vi "test_section_daqmx_task.vi"(8 "error in":errorcluster, 9 "Test Section Physical Channels":T1={"Vapor Mass Flow Current"="cDAQ1Mod1/ai10", "Vapor Line Density Current"="cDAQ1Mod1/ai11", "Liquid Mass Flow Current"="cDAQ1Mod1/ai8", "Liquid Line Density Current"="cDAQ1Mod1/ai9", "Vapor Tank Pressure"="cDAQ1Mod1/ai3", "Liquid Tank Pressure"="cDAQ1Mod1/ai6", "Separator Pressure"="cDAQ1Mod1/ai2", "Liquid Inlet Pressure"="cDAQ1Mod1/ai4", "Dev Section Pressure"="cDAQ1Mod1/ai0", "Vapor Tank Temperature"="cDAQ1Mod1/ai1", "Vapor Inlet Temperature"="cDAQ1Mod6/ai2", "Liquid Tank Temperature"="cDAQ1Mod6/ai0", "Liquid Inlet Temperature"="cDAQ1Mod6/ai3", "Separator Temperature"="cDAQ1Mod6/ai4", "Lower Test Section Pressure"="cDAQ1Mod6/ai1", "Lower Test Section Temperature"="cDAQ1Mod1/ai5", "Top Heater Temperature"="cDAQ1Mod6/ai5", "Bottom Heater Temperature"="cDAQ1Mod6/ai6", "Pressure Drop"="cDAQ1Mod1/ai12", "Upper Test Section Temperature"="cDAQ1Mod1/ai12", "Upper Test Section Pressure"="cDAQ1Mod6/ai9", "Condenser Top Temperature"="cDAQ1Mod1/ai7", "Condenser Bottom Temperature"="cDAQ1Mod6/ai8", "Evaporator Top Temperature"="cDAQ1Mod6/ai10", "Evaporator Bottom Temperature"="cDAQ1Mod6/ai11", "Test Section Window 3-4 Pressure"="cDAQ1Mod6/ai12"}, 10 "sampling rate":dbl, 11 "number of samples":i32) -> (0 "error out":errorcluster, 3 "task out":refnum<k21>)   [LabVIEW 2015]
uses:
  <vilib>/DAQmx/create/channels.llb/DAQmx Create Channel (TEDS-AI-Current-Basic).vi
  <vilib>/DAQmx/create/channels.llb/DAQmx Create Channel (AI-Current-Basic).vi
  <vilib>/DAQmx/create/channels.llb/DAQmx Create Channel (AI-Voltage-Basic).vi
  <vilib>/DAQmx/create/channels.llb/DAQmx Create Channel (TEDS-AI-Voltage-Basic).vi
  <vilib>/DAQmx/create/channels.llb/DAQmx Create Channel (TEDS-AI-Temperature-Thermocouple).vi
  <vilib>/DAQmx/create/channels.llb/DAQmx Create Channel (AI-Temperature-Thermocouple).vi
  <resource>/objmgr/daqmx.rc
  <vilib>/DAQmx/configure/timing.llb/DAQmx Timing (Sample Clock).vi
  Input Channel Lists/test_section_physical_channels.ctl
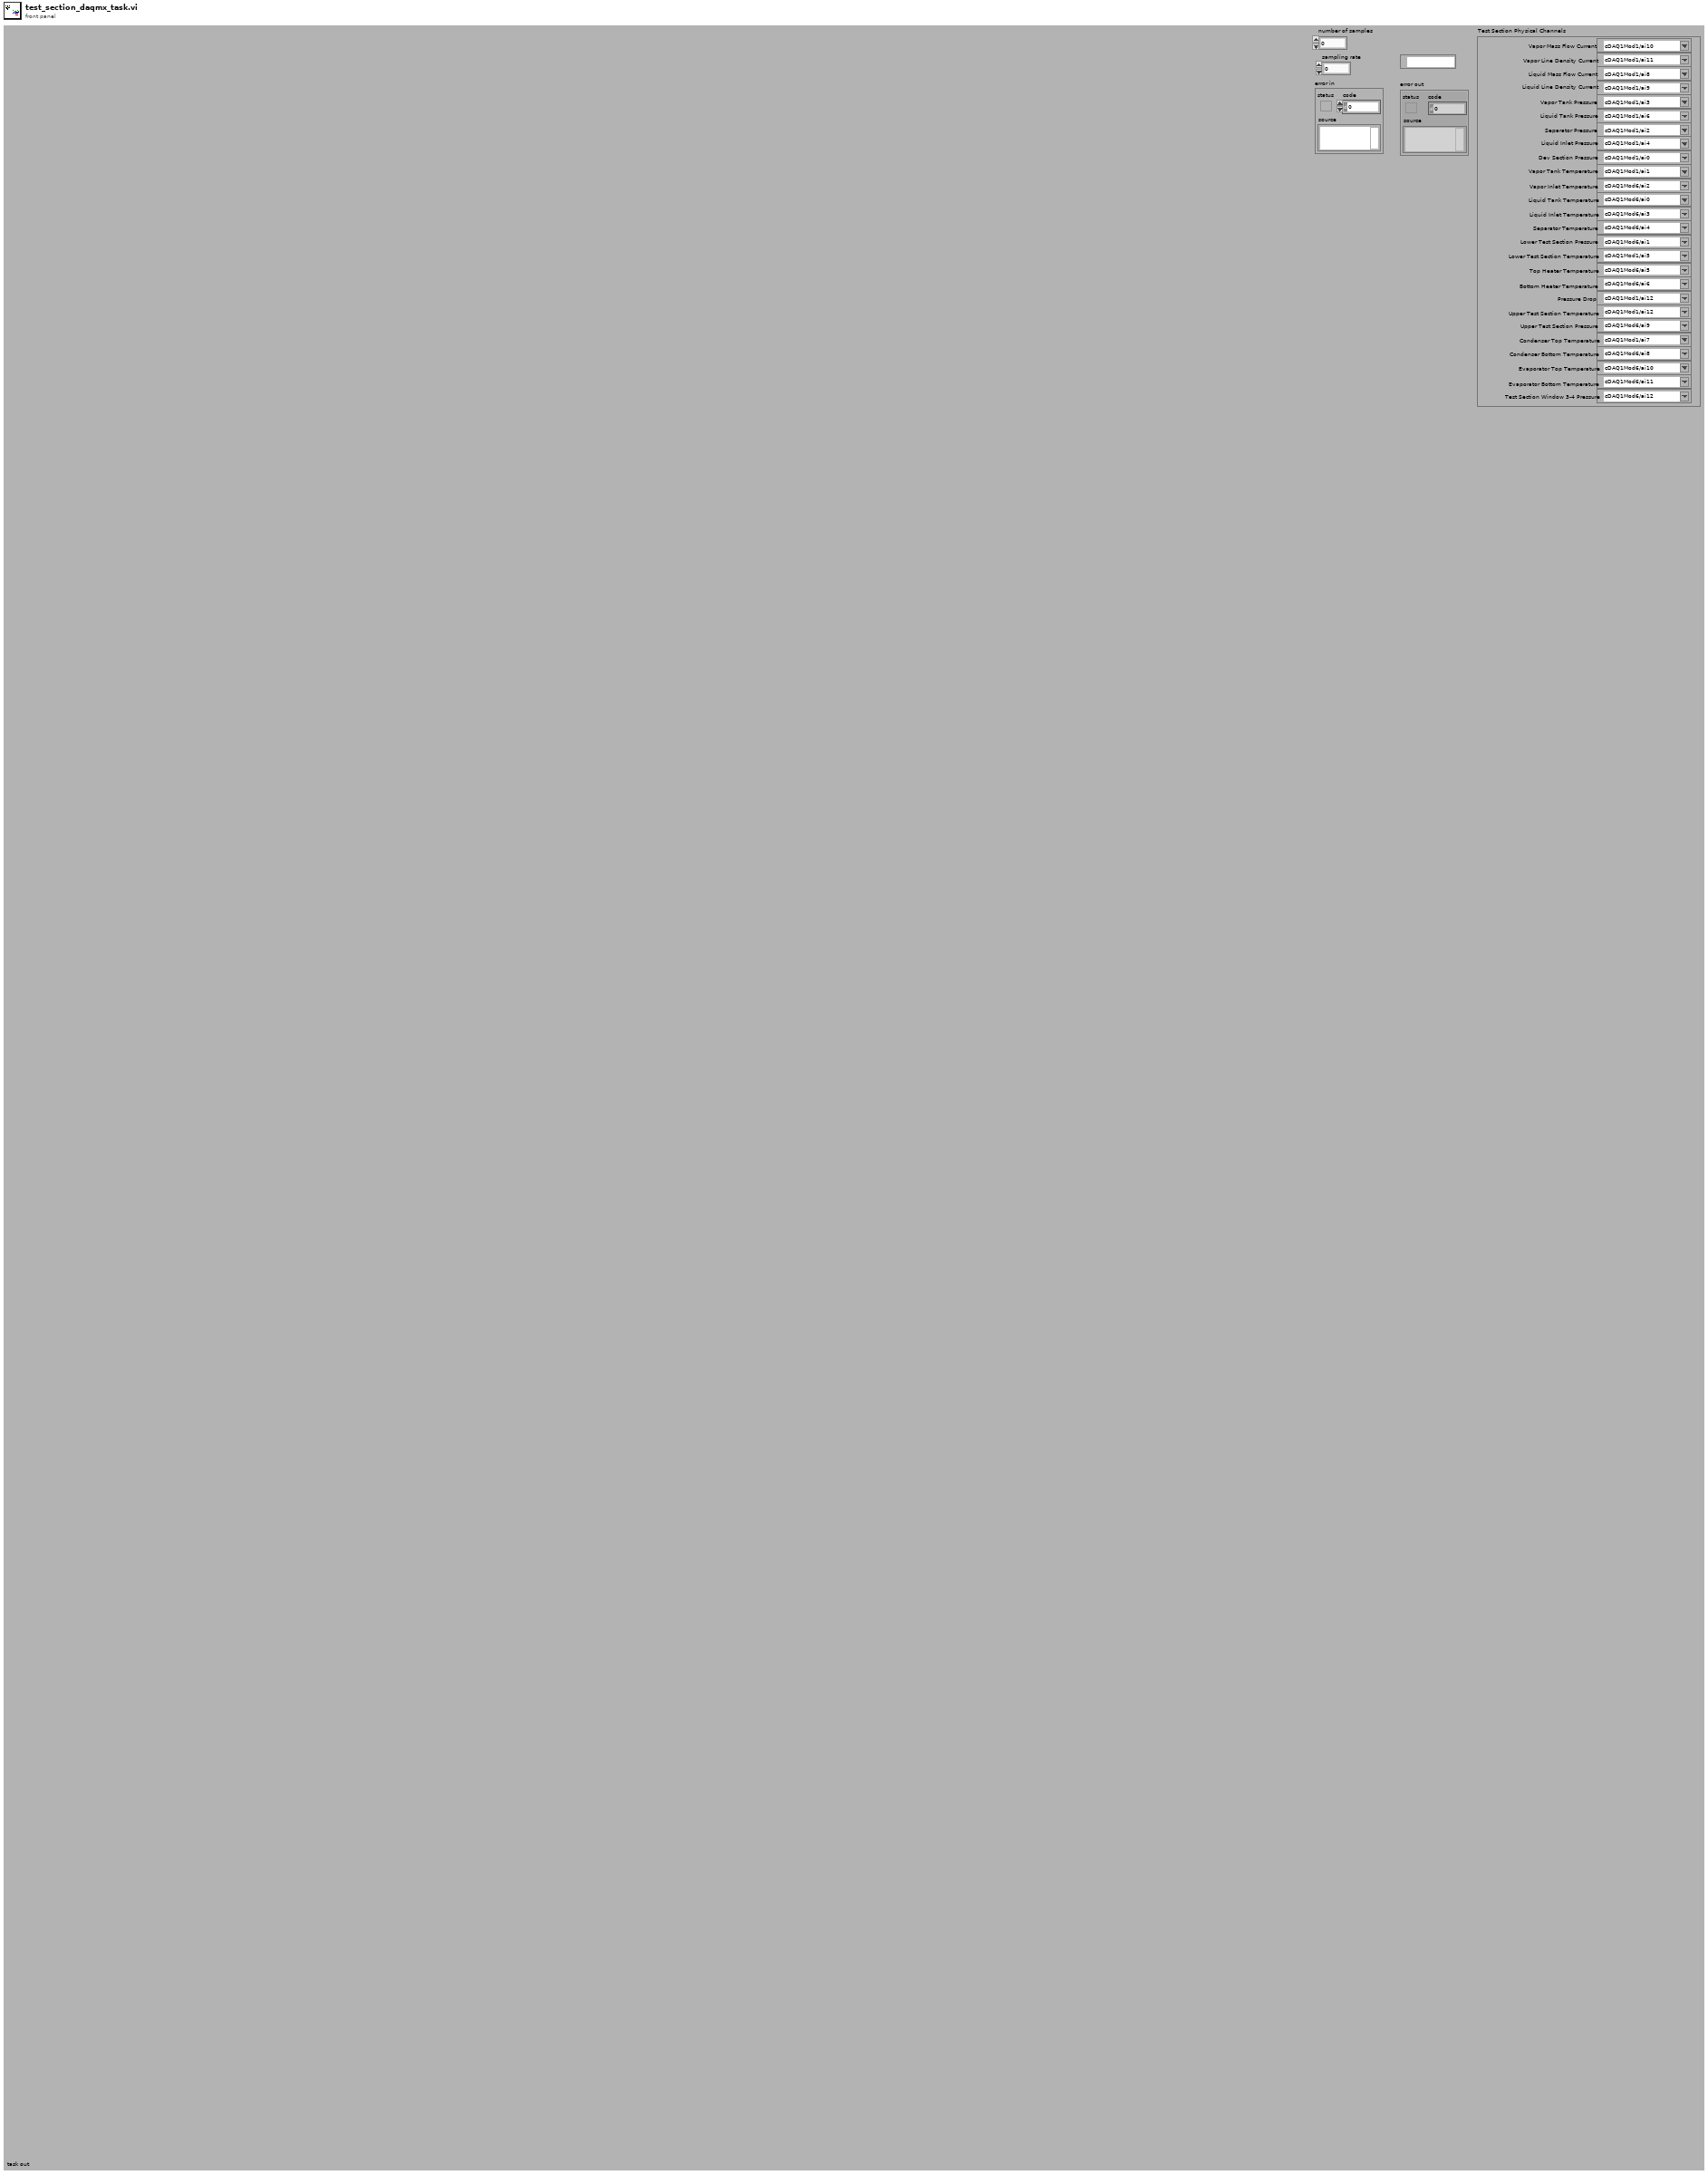
[diagram p1: front panel]
types:
  T1 = typedef "test_section_physical_channels.ctl" = cluster{"Vapor Mass Flow Current":tag, "Vapor Line Density Current":tag, "Liquid Mass Flow Current":tag, "Liquid Line Density Current":tag, "Vapor Tank Pressure":tag, "Liquid Tank Pressure":tag, "Separator Pressure":tag, "Liquid Inlet Pressure":tag, "Dev Section Pressure":tag, "Vapor Tank Temperature":tag, "Vapor Inlet Temperature":tag, "Liquid Tank Temperature":tag, "Liquid Inlet Temperature":tag, "Separator Temperature":tag, "Lower Test Section Pressure":tag, "Lower Test Section Temperature":tag, "Top Heater Temperature":tag, "Bottom Heater Temperature":tag, "Pressure Drop":tag, "Upper Test Section Temperature":tag, "Upper Test Section Pressure":tag, "Condenser Top Temperature":tag, "Condenser Bottom Temperature":tag, "Evaporator Top Temperature":tag, "Evaporator Bottom Temperature":tag, "Test Section Window 3-4 Pressure":tag}
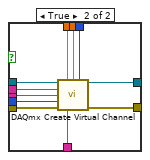
[diagram p2: hidden frame]
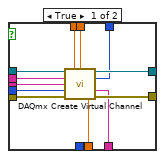
[diagram p3: hidden frame]
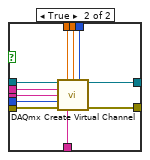
[diagram p4: hidden frame]
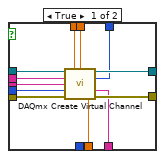
[diagram p5: hidden frame]
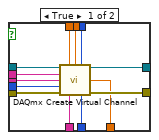
[diagram p6: hidden frame]
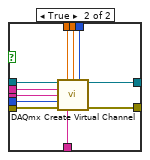
[diagram p7: hidden frame]
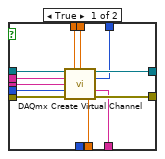
[diagram p8: hidden frame]
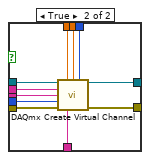
[diagram p9: hidden frame]
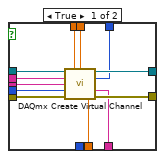
[diagram p10: hidden frame]
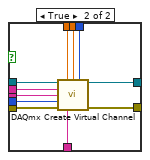
[diagram p11: hidden frame]
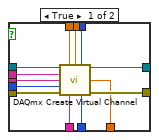
[diagram p12: hidden frame]
diagram:
  w42 = 10123 items=["Finite Samples"=10178, "Continuous Samples"=10123, "Hardware Timed Single Point"=12522]  # sample mode
  w47 = i32[] [10195] items=["High Resolution"=10195, "High Speed"=14712, "Best 50 Hz Rejection"=14713, "Best 60 Hz Rejection"=14714]  # ADCTimingMode
  w49 = string[] ["Test Section Window 3-4 P"]  # ActiveChan
  w51 = i32[] [10164, 10164, 10164, 10164] items=["None"=10230, "Once"=10244, "Every Sample"=10164]  # AutoZeroMode
  w53 = string[] ["Condenser Top Temp", "Condenser Bottom Temp", "Evaporator top temp", "Evaporator Bottom Temp"]  # ActiveChan
  w55 = i32[] [10195] items=["High Resolution"=10195, "High Speed"=14712, "Best 50 Hz Rejection"=14713, "Best 60 Hz Rejection"=14714]  # ADCTimingMode
  w57 = string[] ["Upper TS Pressure"]  # ActiveChan
  w59 = i32[] [10164] items=["None"=10230, "Once"=10244, "Every Sample"=10164]  # AutoZeroMode
  w61 = string[] ["Upper test section Temp"]  # ActiveChan
  w63 = i32[] [10195] items=["High Resolution"=10195, "High Speed"=14712, "Best 50 Hz Rejection"=14713, "Best 60 Hz Rejection"=14714]  # ADCTimingMode
  w65 = string[] ["Pressure Drop"]  # ActiveChan
  w67 = i32[] [10164, 10164, 10164] items=["None"=10230, "Once"=10244, "Every Sample"=10164]  # AutoZeroMode
  w69 = string[] ["Lower Test Section Temp", "Top Heater Temp", "Bottom Heater Temp"]  # ActiveChan
  w71 = i32[] [10195] items=["High Resolution"=10195, "High Speed"=14712, "Best 50 Hz Rejection"=14713, "Best 60 Hz Rejection"=14714]  # ADCTimingMode
  w73 = string[] ["Lower Test Section Pressure"]  # ActiveChan
  w75 = i32[] [10164, 10164, 10164, 10164, 10164] items=["None"=10230, "Once"=10244, "Every Sample"=10164]  # AutoZeroMode
  w77 = string[] ["Vapor Tank Temp", "Vapor Inlet Temp", "Liquid Tank Temp", "Liquid Inlet Temp", "Separator Temp"]  # ActiveChan
  w79 = i32[] [10195, 10195, 10195, 10195, 10195, 10195, 10195, 10195, 10195] items=["High Resolution"=10195, "High Speed"=14712, "Best 50 Hz Rejection"=14713, "Best 60 Hz Rejection"=14714]  # ADCTimingMode
  w81 = string[] ["Vapor Mass Flow Current", "Vapor Line Density Current", "Liquid Mass Flow Current", "Liquid Line Density Current", "Vapor Tank Pressure", "Liquid Tank Pressure", "Separator Pressure", "Liquid Inlet Pressure", "Dev Section Pressure"]  # ActiveChan
  w82 = bool[] [FALSE, FALSE]  # TEDS channel
  w86 = string[] ["", ""]  # custom scale name
  w85 = i32[] [10348, 10348] items=["Volts"=10348, "From TEDS"=12516, "From Custom Scale"=10065]  # units
  w84 = string[] ["Evaporator Bottom Temp", "Test Section Window 3-4 P"]  # channel name
  (unwired) string[] ["cDAQ1Mod6/ai12", "cDAQ1Mod1/ai6"]  # physical channel
  w87 = dbl[] [0.078125, 5.0]  # maximum value
  w88 = dbl[] [-0.078125, 1.0]  # minimum value
  w89 = i32[] [10106, 10106] items=["default"=-1, "RSE"=10083, "NRSE"=10078, "Differential"=10106, "Pseudodifferential"=12529]  # input terminal configuration
  w91 = bool[] [FALSE]  # TEDS channel
  w93 = dbl[] [25.0]  # cjc value
  w92 = string[] [""]  # cjc channel
  w98 = i32[] [10086] items=["J"=10072, "K"=10073, "N"=10077, "R"=10082, "S"=10085, "T"=10086, "B"=10047, "E"=10055]  # thermocouple type
  w97 = i32[] [10143] items=["deg C"=10143, "deg F"=10144, "Kelvins"=10325, "deg R"=10145, "From Custom Scale"=10065]  # units
  w96 = string[] ["Evaporator top temp"]  # channel name
  (unwired) string[] ["cDAQ1Mod6/ai11"]  # physical channel
  w99 = dbl[] [100.0]  # maximum value
  w100 = dbl[] [0.0]  # minimum value
  w94 = u32[] [10200] items=["Internal"=10200, "Constant Value"=10116, "Channel"=10113]  # cjc source
  w102 = bool[] [FALSE, FALSE, FALSE]  # TEDS channel
  w106 = string[] ["", "", ""]  # custom scale name
  w105 = i32[] [10348, 10348, 10348] items=["Volts"=10348, "From TEDS"=12516, "From Custom Scale"=10065]  # units
  w104 = string[] ["Upper TS Pressure", "Condenser Top Temp", "Condenser Bottom Temp"]  # channel name
  (unwired) string[] ["cDAQ1Mod1/ai7", "cDAQ1Mod6/ai8", "cDAQ1Mod6/ai10"]  # physical channel
  w107 = dbl[] [10.0, 0.078125, 0.078125]  # maximum value
  w108 = dbl[] [-10.0, -0.078125, -0.078125]  # minimum value
  w109 = i32[] [10106, 10106, 10106] items=["default"=-1, "RSE"=10083, "NRSE"=10078, "Differential"=10106, "Pseudodifferential"=12529]  # input terminal configuration
  w111 = bool[] [FALSE]  # TEDS channel
  w113 = dbl[] [25.0]  # cjc value
  w112 = string[] [""]  # cjc channel
  w118 = i32[] [10086] items=["J"=10072, "K"=10073, "N"=10077, "R"=10082, "S"=10085, "T"=10086, "B"=10047, "E"=10055]  # thermocouple type
  w117 = i32[] [10143] items=["deg C"=10143, "deg F"=10144, "Kelvins"=10325, "deg R"=10145, "From Custom Scale"=10065]  # units
  w116 = string[] ["Upper test section Temp"]  # channel name
  (unwired) string[] ["cDAQ1Mod6/ai9"]  # physical channel
  w119 = dbl[] [100.0]  # maximum value
  w120 = dbl[] [0.0]  # minimum value
  w114 = u32[] [10200] items=["Internal"=10200, "Constant Value"=10116, "Channel"=10113]  # cjc source
  w122 = bool[] [FALSE]  # TEDS channel
  w124 = i32[] [10200] items=["Internal"=10200, "External"=10167]  # shunt resistor location
  w123 = dbl[] [34.01]  # shunt resistor value
  w128 = string[] [""]  # custom scale name
  w127 = i32[] [10342] items=["Amps"=10342, "From TEDS"=12516, "From Custom Scale"=10065]  # units
  w126 = string[] ["Pressure Drop"]  # channel name
  (unwired) string[] ["cDAQ1Mod1/ai12"]  # physical channel
  w129 = dbl[] [0.02]  # maximum value
  w130 = dbl[] [-0.02]  # minimum value
  w131 = i32[] [10083] items=["default"=-1, "RSE"=10083, "NRSE"=10078, "Differential"=10106, "Pseudodifferential"=12529]  # input terminal configuration
  w133 = bool[] [FALSE, FALSE]  # TEDS channel
  w137 = string[] ["", ""]  # custom scale name
  w136 = i32[] [10348, 10348] items=["Volts"=10348, "From TEDS"=12516, "From Custom Scale"=10065]  # units
  w135 = string[] ["Top Heater Temp", "Bottom Heater Temp"]  # channel name
  (unwired) string[] ["cDAQ1Mod6/ai6", "cDAQ1Mod6/ai7"]  # physical channel
  w138 = dbl[] [0.078125, 0.078125]  # maximum value
  w139 = dbl[] [-0.078125, -0.078125]  # minimum value
  w140 = i32[] [10106, 10106] items=["default"=-1, "RSE"=10083, "NRSE"=10078, "Differential"=10106, "Pseudodifferential"=12529]  # input terminal configuration
  w142 = bool[] [FALSE]  # TEDS channel
  w144 = dbl[] [25.0]  # cjc value
  w143 = string[] [""]  # cjc channel
  w149 = i32[] [10086] items=["J"=10072, "K"=10073, "N"=10077, "R"=10082, "S"=10085, "T"=10086, "B"=10047, "E"=10055]  # thermocouple type
  w148 = i32[] [10143] items=["deg C"=10143, "deg F"=10144, "Kelvins"=10325, "deg R"=10145, "From Custom Scale"=10065]  # units
  w147 = string[] ["Lower Test Section Temp"]  # channel name
  (unwired) string[] ["cDAQ1Mod6/ai5"]  # physical channel
  w150 = dbl[] [100.0]  # maximum value
  w151 = dbl[] [0.0]  # minimum value
  w145 = u32[] [10200] items=["Internal"=10200, "Constant Value"=10116, "Channel"=10113]  # cjc source
  w153 = bool[] [FALSE]  # TEDS channel
  w157 = string[] [""]  # custom scale name
  w156 = i32[] [10348] items=["Volts"=10348, "From TEDS"=12516, "From Custom Scale"=10065]  # units
  w155 = string[] ["Lower Test Section Pressure"]  # channel name
  (unwired) string[] ["cDAQ1Mod1/ai5"]  # physical channel
  w158 = dbl[] [5.0]  # maximum value
  w159 = dbl[] [0.0]  # minimum value
  w160 = i32[] [10106] items=["default"=-1, "RSE"=10083, "NRSE"=10078, "Differential"=10106, "Pseudodifferential"=12529]  # input terminal configuration
  w162 = bool[] [FALSE, FALSE, FALSE, FALSE, FALSE]  # TEDS channel
  w164 = dbl[] [25.0, 25.0, 25.0, 25.0, 25.0]  # cjc value
  w163 = string[] ["", "", "", "", ""]  # cjc channel
  w169 = i32[] [10086, 10086, 10086, 10086, 10072] items=["J"=10072, "K"=10073, "N"=10077, "R"=10082, "S"=10085, "T"=10086, "B"=10047, "E"=10055]  # thermocouple type
  w168 = i32[] [10143, 10143, 10143, 10143, 10143] items=["deg C"=10143, "deg F"=10144, "Kelvins"=10325, "deg R"=10145, "From Custom Scale"=10065]  # units
  w167 = string[] ["Vapor Tank Temp", "Vapor Inlet Temp", "Liquid Tank Temp", "Liquid Inlet Temp", "Separator Temp"]  # channel name
  (unwired) string[] ["cDAQ1Mod6/ai2", "cDAQ1Mod6/ai0", "cDAQ1Mod6/ai3", "cDAQ1Mod6/ai4", "cDAQ1Mod6/ai1"]  # physical channel
  w170 = dbl[] [100.0, 100.0, 100.0, 100.0, 100.0]  # maximum value
  w171 = dbl[] [0.0, 0.0, 0.0, 0.0, 0.0]  # minimum value
  w165 = u32[] [10200, 10200, 10200, 10200, 10200] items=["Internal"=10200, "Constant Value"=10116, "Channel"=10113]  # cjc source
  w173 = bool[] [FALSE, FALSE, FALSE, FALSE, FALSE]  # TEDS channel
  w177 = string[] ["", "", "", "", ""]  # custom scale name
  w176 = i32[] [10348, 10348, 10348, 10348, 10348] items=["Volts"=10348, "From TEDS"=12516, "From Custom Scale"=10065]  # units
  w175 = string[] ["Vapor Tank Pressure", "Liquid Tank Pressure", "Separator Pressure", "Liquid Inlet Pressure", "Dev Section Pressure"]  # channel name
  (unwired) string[] ["cDAQ1Mod1/ai3", "cDAQ1Mod1/ai2", "cDAQ1Mod1/ai4", "cDAQ1Mod1/ai0", "cDAQ1Mod1/ai1"]  # physical channel
  w178 = dbl[] [5.5, 5.0, 5.5, 5.5, 5.0]  # maximum value
  w179 = dbl[] [0.5, 0.0, 0.5, 0.5, 0.0]  # minimum value
  w180 = i32[] [10106, 10106, 10106, 10106, 10106] items=["default"=-1, "RSE"=10083, "NRSE"=10078, "Differential"=10106, "Pseudodifferential"=12529]  # input terminal configuration
  w182 = bool[] [FALSE, FALSE, FALSE, FALSE]  # TEDS channel
  w184 = i32[] [10200, 10200, 10200, 10200] items=["Internal"=10200, "External"=10167]  # shunt resistor location
  w183 = dbl[] [34.01, 34.01, 34.01, 34.01]  # shunt resistor value
  w188 = string[] ["", "", "", ""]  # custom scale name
  w187 = i32[] [10342, 10342, 10342, 10342] items=["Amps"=10342, "From TEDS"=12516, "From Custom Scale"=10065]  # units
  w186 = string[] ["Vapor Mass Flow Current", "Vapor Line Density Current", "Liquid Mass Flow Current", "Liquid Line Density Current"]  # channel name
  (unwired) string[] ["cDAQ1Mod1/ai10", "cDAQ1Mod1/ai11", "cDAQ1Mod1/ai8", "cDAQ1Mod1/ai9"]  # physical channel
  w189 = dbl[] [0.02, 0.02, 0.02, 0.02]  # maximum value
  w190 = dbl[] [-0.02, -0.02, -0.02, -0.02]  # minimum value
  w191 = i32[] [10083, 10083, 10083, 10083] items=["default"=-1, "RSE"=10083, "NRSE"=10078, "Differential"=10106, "Pseudodifferential"=12529]  # input terminal configuration
  w193 = FALSE  # auto cleanup
  n1 = Unbundle By Name("Test Section Physical Channels") -> ("Vapor Mass Flow Current"=w38:tag, "Vapor Line Density Current"=w37:tag, "Liquid Mass Flow Current"=w36:tag, "Liquid Line Density Current"=w35:tag)
  n2 = Build Array(w38, w37, w36, w35) -> (w34:tag[])
  n3 = call <vilib>:"DAQmx Create Task.vi"("new task name"="MainLoop", "auto cleanup"=w193, "error in"="error in") -> ("task out"=w192:refnum<k21>, "error out"=w194:errorcluster)  [unwired: 11 in]
  n4 = for {
    tunnel: w192 -> [w206]
    tunnel: w191 -> [w209] mode=indexing
    tunnel: w190 -> [w208] mode=indexing
    tunnel: w189 -> [w207] mode=indexing
    tunnel: w188 -> [w202] mode=indexing
    tunnel: w187 -> [w199] mode=indexing
    tunnel: w186 -> [w201] mode=indexing
    tunnel: w34 -> [w200] mode=indexing
    tunnel: [w204] -> w181
    tunnel: w184 -> [w198] mode=indexing
    tunnel: w183 -> [w197] mode=indexing
    shift-right: [w203] -> w185
    shift-left: w194 -> [w205]
    tunnel: w182 -> [w196] mode=indexing
    n5 = case shown="False" w196 {
      tunnel: w209 -> [w222 w235]
      tunnel: w208 -> [w221 w234]
      tunnel: w207 -> [w220 w233]
      tunnel: w206 -> [w219 w232]
      tunnel: w205 -> [w218 w231]
      tunnel: [w217 w230] -> w204
      tunnel: [w216 w229] -> w203
      tunnel: w202 -> [w215 w228]
      tunnel: w201 -> [w214 w227]
      tunnel: w200 -> [w213 w226]
      tunnel: w199 -> [w212 w225]
      tunnel: w198 -> [w211 w224]
      tunnel: w197 -> [w210 w223]
      frame True {
        n6 = call-poly <vilib>:"DAQmx Create Virtual Channel.vi"("task in"=w219, "maximum value"=w220, "minimum value"=w221, "input terminal configuration"=w222, "physical channels"=w213, "name to assign"=w214, "external shunt resistor value"=w210, "units"=w212, "error in"=w218, "custom scale name"=w215, "shunt resistor location"=w211) -> ("task out"=w217:refnum<k21>, "error out"=w216:errorcluster)  [unwired: 3 in]
      }
      frame False {
        n7 = call-poly <vilib>:"DAQmx Create Virtual Channel.vi"("task in"=w232, "maximum value"=w233, "minimum value"=w234, "input terminal configuration"=w235, "physical channels"=w226, "name to assign"=w227, "external shunt resistor value"=w223, "units"=w225, "error in"=w231, "custom scale name"=w228, "shunt resistor location"=w224) -> ("task out"=w230:refnum<k21>, "error out"=w229:errorcluster)  [unwired: 3 in]
      }
    }
  }
  n8 = Unbundle By Name("Test Section Physical Channels") -> ("Vapor Tank Pressure"=w30:tag, "Liquid Tank Pressure"=w31:tag, "Separator Pressure"=w32:tag, "Liquid Inlet Pressure"=w33:tag, "Dev Section Pressure"=w24:tag)
  n9 = Build Array(w30, w31, w32, w33, w24) -> (w23:tag[])
  n10 = for {
    tunnel: w181 -> [w244]
    tunnel: w180 -> [w245] mode=indexing
    tunnel: w179 -> [w246] mode=indexing
    tunnel: w178 -> [w247] mode=indexing
    tunnel: w177 -> [w237] mode=indexing
    tunnel: w176 -> [w238] mode=indexing
    tunnel: w175 -> [w240] mode=indexing
    tunnel: w23 -> [w239] mode=indexing
    tunnel: [w242] -> w172
    shift-right: [w241] -> w174
    shift-left: w185 -> [w243]
    tunnel: w173 -> [w236] mode=indexing
    n11 = case shown="False" w236 {
      tunnel: w247 -> [w258 w263]
      tunnel: w246 -> [w257 w264]
      tunnel: w245 -> [w256 w265]
      tunnel: w244 -> [w255 w269]
      tunnel: w243 -> [w254 w268]
      tunnel: [w253 w266] -> w242
      tunnel: [w252 w267] -> w241
      tunnel: w240 -> [w251 w261]
      tunnel: w239 -> [w250 w262]
      tunnel: w238 -> [w249 w260]
      tunnel: w237 -> [w248 w259]
      frame False {
        n12 = call-poly <vilib>:"DAQmx Create Virtual Channel.vi"("task in"=w255, "maximum value"=w258, "minimum value"=w257, "input terminal configuration"=w256, "physical channels"=w250, "name to assign"=w251, "units"=w249, "error in"=w254, "custom scale name"=w248) -> ("task out"=w253:refnum<k21>, "error out"=w252:errorcluster)  [unwired: 5 in]
      }
      frame True {
        n13 = call-poly <vilib>:"DAQmx Create Virtual Channel.vi"("task in"=w269, "maximum value"=w263, "minimum value"=w264, "input terminal configuration"=w265, "physical channels"=w262, "name to assign"=w261, "units"=w260, "error in"=w268, "custom scale name"=w259) -> ("task out"=w266:refnum<k21>, "error out"=w267:errorcluster)  [unwired: 5 in]
      }
    }
  }
  n14 = Unbundle By Name("Test Section Physical Channels") -> ("Vapor Tank Temperature"=w29:tag, "Vapor Inlet Temperature"=w28:tag, "Liquid Tank Temperature"=w27:tag, "Liquid Inlet Temperature"=w26:tag, "Separator Temperature"=w22:tag)
  n15 = Build Array(w29, w28, w27, w26, w22) -> (w21:tag[])
  n16 = for {
    tunnel: w172 -> [w281]
    tunnel: w171 -> [w282] mode=indexing
    tunnel: w170 -> [w283] mode=indexing
    tunnel: w169 -> [w271] mode=indexing
    tunnel: w168 -> [w275] mode=indexing
    tunnel: w167 -> [w277] mode=indexing
    tunnel: w21 -> [w276] mode=indexing
    tunnel: [w279] -> w161
    tunnel: w165 -> [w274] mode=indexing
    tunnel: w164 -> [w273] mode=indexing
    tunnel: w163 -> [w272] mode=indexing
    shift-right: [w278] -> w166
    shift-left: w174 -> [w280]
    tunnel: w162 -> [w270] mode=indexing
    n17 = case shown="False" w270 {
      tunnel: w283 -> [w295 w308]
      tunnel: w282 -> [w294 w307]
      tunnel: w281 -> [w293 w306]
      tunnel: w280 -> [w292 w305]
      tunnel: [w291 w304] -> w279
      tunnel: [w290 w303] -> w278
      tunnel: w277 -> [w289 w302]
      tunnel: w276 -> [w288 w301]
      tunnel: w275 -> [w287 w300]
      tunnel: w274 -> [w286 w299]
      tunnel: w273 -> [w285 w298]
      tunnel: w272 -> [w284 w297]
      tunnel: w271 -> [_ w296]
      frame True {
        n18 = call-poly <vilib>:"DAQmx Create Virtual Channel.vi"("task in"=w293, "maximum value"=w295, "minimum value"=w294, "physical channels"=w288, "cjc source"=w286, "name to assign"=w289, "units"=w287, "cjc channel"=w284, "error in"=w292, "cjc value"=w285) -> ("task out"=w291:refnum<k21>, "error out"=w290:errorcluster)  [unwired: 4 in]
      }
      frame False {
        n19 = call-poly <vilib>:"DAQmx Create Virtual Channel.vi"("task in"=w306, "maximum value"=w308, "minimum value"=w307, "physical channels"=w301, "cjc source"=w299, "name to assign"=w302, "units"=w300, "cjc channel"=w297, "error in"=w305, "thermocouple type"=w296, "cjc value"=w298) -> ("task out"=w304:refnum<k21>, "error out"=w303:errorcluster)  [unwired: 3 in]
      }
    }
  }
  n20 = Unbundle By Name("Test Section Physical Channels") -> ("Lower Test Section Pressure"=w25:tag)
  n21 = Build Array(w25) -> (w20:tag[])
  n22 = Unbundle By Name("Test Section Physical Channels") -> ("Lower Test Section Temperature"=w19:tag)
  n23 = for {
    tunnel: w161 -> [w317]
    tunnel: w160 -> [w318] mode=indexing
    tunnel: w159 -> [w319] mode=indexing
    tunnel: w158 -> [w320] mode=indexing
    tunnel: w157 -> [w310] mode=indexing
    tunnel: w156 -> [w311] mode=indexing
    tunnel: w155 -> [w313] mode=indexing
    tunnel: w20 -> [w312] mode=indexing
    tunnel: [w315] -> w152
    shift-right: [w314] -> w154
    shift-left: w166 -> [w316]
    tunnel: w153 -> [w309] mode=indexing
    n24 = case shown="False" w309 {
      tunnel: w320 -> [w331 w336]
      tunnel: w319 -> [w330 w337]
      tunnel: w318 -> [w329 w338]
      tunnel: w317 -> [w328 w342]
      tunnel: w316 -> [w327 w341]
      tunnel: [w326 w339] -> w315
      tunnel: [w325 w340] -> w314
      tunnel: w313 -> [w324 w334]
      tunnel: w312 -> [w323 w335]
      tunnel: w311 -> [w322 w333]
      tunnel: w310 -> [w321 w332]
      frame False {
        n25 = call-poly <vilib>:"DAQmx Create Virtual Channel.vi"("task in"=w328, "maximum value"=w331, "minimum value"=w330, "input terminal configuration"=w329, "physical channels"=w323, "name to assign"=w324, "units"=w322, "error in"=w327, "custom scale name"=w321) -> ("task out"=w326:refnum<k21>, "error out"=w325:errorcluster)  [unwired: 5 in]
      }
      frame True {
        n26 = call-poly <vilib>:"DAQmx Create Virtual Channel.vi"("task in"=w342, "maximum value"=w336, "minimum value"=w337, "input terminal configuration"=w338, "physical channels"=w335, "name to assign"=w334, "units"=w333, "error in"=w341, "custom scale name"=w332) -> ("task out"=w339:refnum<k21>, "error out"=w340:errorcluster)  [unwired: 5 in]
      }
    }
  }
  n27 = Build Array(w19) -> (w18:tag[])
  n28 = for {
    tunnel: w152 -> [w354]
    tunnel: w151 -> [w355] mode=indexing
    tunnel: w150 -> [w356] mode=indexing
    tunnel: w149 -> [w344] mode=indexing
    tunnel: w148 -> [w348] mode=indexing
    tunnel: w147 -> [w350] mode=indexing
    tunnel: w18 -> [w349] mode=indexing
    tunnel: [w352] -> w141
    tunnel: w145 -> [w347] mode=indexing
    tunnel: w144 -> [w346] mode=indexing
    tunnel: w143 -> [w345] mode=indexing
    shift-right: [w351] -> w146
    shift-left: w154 -> [w353]
    tunnel: w142 -> [w343] mode=indexing
    n29 = case shown="False" w343 {
      tunnel: w356 -> [w368 w381]
      tunnel: w355 -> [w367 w380]
      tunnel: w354 -> [w366 w379]
      tunnel: w353 -> [w365 w378]
      tunnel: [w364 w377] -> w352
      tunnel: [w363 w376] -> w351
      tunnel: w350 -> [w362 w375]
      tunnel: w349 -> [w361 w374]
      tunnel: w348 -> [w360 w373]
      tunnel: w347 -> [w359 w372]
      tunnel: w346 -> [w358 w371]
      tunnel: w345 -> [w357 w370]
      tunnel: w344 -> [_ w369]
      frame True {
        n30 = call-poly <vilib>:"DAQmx Create Virtual Channel.vi"("task in"=w366, "maximum value"=w368, "minimum value"=w367, "physical channels"=w361, "cjc source"=w359, "name to assign"=w362, "units"=w360, "cjc channel"=w357, "error in"=w365, "cjc value"=w358) -> ("task out"=w364:refnum<k21>, "error out"=w363:errorcluster)  [unwired: 4 in]
      }
      frame False {
        n31 = call-poly <vilib>:"DAQmx Create Virtual Channel.vi"("task in"=w379, "maximum value"=w381, "minimum value"=w380, "physical channels"=w374, "cjc source"=w372, "name to assign"=w375, "units"=w373, "cjc channel"=w370, "error in"=w378, "thermocouple type"=w369, "cjc value"=w371) -> ("task out"=w377:refnum<k21>, "error out"=w376:errorcluster)  [unwired: 3 in]
      }
    }
  }
  n32 = Unbundle By Name("Test Section Physical Channels") -> ("Top Heater Temperature"=w13:tag, "Bottom Heater Temperature"=w17:tag)
  n33 = Build Array(w13, w17) -> (w16:tag[])
  n34 = for {
    tunnel: w141 -> [w390]
    tunnel: w140 -> [w391] mode=indexing
    tunnel: w139 -> [w392] mode=indexing
    tunnel: w138 -> [w393] mode=indexing
    tunnel: w137 -> [w383] mode=indexing
    tunnel: w136 -> [w384] mode=indexing
    tunnel: w135 -> [w386] mode=indexing
    tunnel: w16 -> [w385] mode=indexing
    tunnel: [w388] -> w132
    shift-right: [w387] -> w134
    shift-left: w146 -> [w389]
    tunnel: w133 -> [w382] mode=indexing
    n35 = case shown="False" w382 {
      tunnel: w393 -> [w404 w409]
      tunnel: w392 -> [w403 w410]
      tunnel: w391 -> [w402 w411]
      tunnel: w390 -> [w401 w415]
      tunnel: w389 -> [w400 w414]
      tunnel: [w399 w412] -> w388
      tunnel: [w398 w413] -> w387
      tunnel: w386 -> [w397 w407]
      tunnel: w385 -> [w396 w408]
      tunnel: w384 -> [w395 w406]
      tunnel: w383 -> [w394 w405]
      frame False {
        n36 = call-poly <vilib>:"DAQmx Create Virtual Channel.vi"("task in"=w401, "maximum value"=w404, "minimum value"=w403, "input terminal configuration"=w402, "physical channels"=w396, "name to assign"=w397, "units"=w395, "error in"=w400, "custom scale name"=w394) -> ("task out"=w399:refnum<k21>, "error out"=w398:errorcluster)  [unwired: 5 in]
      }
      frame True {
        n37 = call-poly <vilib>:"DAQmx Create Virtual Channel.vi"("task in"=w415, "maximum value"=w409, "minimum value"=w410, "input terminal configuration"=w411, "physical channels"=w408, "name to assign"=w407, "units"=w406, "error in"=w414, "custom scale name"=w405) -> ("task out"=w412:refnum<k21>, "error out"=w413:errorcluster)  [unwired: 5 in]
      }
    }
  }
  n38 = Unbundle By Name("Test Section Physical Channels") -> ("Pressure Drop"=w15:tag)
  n39 = Build Array(w15) -> (w14:tag[])
  n40 = Unbundle By Name("Test Section Physical Channels") -> ("Upper Test Section Temperature"=w12:tag)
  n41 = for {
    tunnel: w132 -> [w426]
    tunnel: w131 -> [w429] mode=indexing
    tunnel: w130 -> [w428] mode=indexing
    tunnel: w129 -> [w427] mode=indexing
    tunnel: w128 -> [w422] mode=indexing
    tunnel: w127 -> [w419] mode=indexing
    tunnel: w126 -> [w421] mode=indexing
    tunnel: w14 -> [w420] mode=indexing
    tunnel: [w424] -> w121
    tunnel: w124 -> [w418] mode=indexing
    tunnel: w123 -> [w417] mode=indexing
    shift-right: [w423] -> w125
    shift-left: w134 -> [w425]
    tunnel: w122 -> [w416] mode=indexing
    n42 = case shown="False" w416 {
      tunnel: w429 -> [w442 w455]
      tunnel: w428 -> [w441 w454]
      tunnel: w427 -> [w440 w453]
      tunnel: w426 -> [w439 w452]
      tunnel: w425 -> [w438 w451]
      tunnel: [w437 w450] -> w424
      tunnel: [w436 w449] -> w423
      tunnel: w422 -> [w435 w448]
      tunnel: w421 -> [w434 w447]
      tunnel: w420 -> [w433 w446]
      tunnel: w419 -> [w432 w445]
      tunnel: w418 -> [w431 w444]
      tunnel: w417 -> [w430 w443]
      frame True {
        n43 = call-poly <vilib>:"DAQmx Create Virtual Channel.vi"("task in"=w439, "maximum value"=w440, "minimum value"=w441, "input terminal configuration"=w442, "physical channels"=w433, "name to assign"=w434, "external shunt resistor value"=w430, "units"=w432, "error in"=w438, "custom scale name"=w435, "shunt resistor location"=w431) -> ("task out"=w437:refnum<k21>, "error out"=w436:errorcluster)  [unwired: 3 in]
      }
      frame False {
        n44 = call-poly <vilib>:"DAQmx Create Virtual Channel.vi"("task in"=w452, "maximum value"=w453, "minimum value"=w454, "input terminal configuration"=w455, "physical channels"=w446, "name to assign"=w447, "external shunt resistor value"=w443, "units"=w445, "error in"=w451, "custom scale name"=w448, "shunt resistor location"=w444) -> ("task out"=w450:refnum<k21>, "error out"=w449:errorcluster)  [unwired: 3 in]
      }
    }
  }
  n45 = Build Array(w12) -> (w11:tag[])
  n46 = Unbundle By Name("Test Section Physical Channels") -> ("Upper Test Section Pressure"=w10:tag, "Condenser Top Temperature"=w9:tag, "Condenser Bottom Temperature"=w8:tag)
  n47 = for {
    tunnel: w121 -> [w467]
    tunnel: w120 -> [w468] mode=indexing
    tunnel: w119 -> [w469] mode=indexing
    tunnel: w118 -> [w457] mode=indexing
    tunnel: w117 -> [w461] mode=indexing
    tunnel: w116 -> [w463] mode=indexing
    tunnel: w11 -> [w462] mode=indexing
    tunnel: [w465] -> w110
    tunnel: w114 -> [w460] mode=indexing
    tunnel: w113 -> [w459] mode=indexing
    tunnel: w112 -> [w458] mode=indexing
    shift-right: [w464] -> w115
    shift-left: w125 -> [w466]
    tunnel: w111 -> [w456] mode=indexing
    n48 = case shown="False" w456 {
      tunnel: w469 -> [w481 w494]
      tunnel: w468 -> [w480 w493]
      tunnel: w467 -> [w479 w492]
      tunnel: w466 -> [w478 w491]
      tunnel: [w477 w490] -> w465
      tunnel: [w476 w489] -> w464
      tunnel: w463 -> [w475 w488]
      tunnel: w462 -> [w474 w487]
      tunnel: w461 -> [w473 w486]
      tunnel: w460 -> [w472 w485]
      tunnel: w459 -> [w471 w484]
      tunnel: w458 -> [w470 w483]
      tunnel: w457 -> [_ w482]
      frame True {
        n49 = call-poly <vilib>:"DAQmx Create Virtual Channel.vi"("task in"=w479, "maximum value"=w481, "minimum value"=w480, "physical channels"=w474, "cjc source"=w472, "name to assign"=w475, "units"=w473, "cjc channel"=w470, "error in"=w478, "cjc value"=w471) -> ("task out"=w477:refnum<k21>, "error out"=w476:errorcluster)  [unwired: 4 in]
      }
      frame False {
        n50 = call-poly <vilib>:"DAQmx Create Virtual Channel.vi"("task in"=w492, "maximum value"=w494, "minimum value"=w493, "physical channels"=w487, "cjc source"=w485, "name to assign"=w488, "units"=w486, "cjc channel"=w483, "error in"=w491, "thermocouple type"=w482, "cjc value"=w484) -> ("task out"=w490:refnum<k21>, "error out"=w489:errorcluster)  [unwired: 3 in]
      }
    }
  }
  n51 = Build Array(w10, w9, w8) -> (w7:tag[])
  n52 = Unbundle By Name("Test Section Physical Channels") -> ("Evaporator Top Temperature"=w6:tag)
  n53 = for {
    tunnel: w110 -> [w503]
    tunnel: w109 -> [w504] mode=indexing
    tunnel: w108 -> [w505] mode=indexing
    tunnel: w107 -> [w506] mode=indexing
    tunnel: w106 -> [w496] mode=indexing
    tunnel: w105 -> [w497] mode=indexing
    tunnel: w104 -> [w499] mode=indexing
    tunnel: w7 -> [w498] mode=indexing
    tunnel: [w501] -> w101
    shift-right: [w500] -> w103
    shift-left: w115 -> [w502]
    tunnel: w102 -> [w495] mode=indexing
    n54 = case shown="False" w495 {
      tunnel: w506 -> [w517 w522]
      tunnel: w505 -> [w516 w523]
      tunnel: w504 -> [w515 w524]
      tunnel: w503 -> [w514 w528]
      tunnel: w502 -> [w513 w527]
      tunnel: [w512 w525] -> w501
      tunnel: [w511 w526] -> w500
      tunnel: w499 -> [w510 w520]
      tunnel: w498 -> [w509 w521]
      tunnel: w497 -> [w508 w519]
      tunnel: w496 -> [w507 w518]
      frame False {
        n55 = call-poly <vilib>:"DAQmx Create Virtual Channel.vi"("task in"=w514, "maximum value"=w517, "minimum value"=w516, "input terminal configuration"=w515, "physical channels"=w509, "name to assign"=w510, "units"=w508, "error in"=w513, "custom scale name"=w507) -> ("task out"=w512:refnum<k21>, "error out"=w511:errorcluster)  [unwired: 5 in]
      }
      frame True {
        n56 = call-poly <vilib>:"DAQmx Create Virtual Channel.vi"("task in"=w528, "maximum value"=w522, "minimum value"=w523, "input terminal configuration"=w524, "physical channels"=w521, "name to assign"=w520, "units"=w519, "error in"=w527, "custom scale name"=w518) -> ("task out"=w525:refnum<k21>, "error out"=w526:errorcluster)  [unwired: 5 in]
      }
    }
  }
  n57 = Build Array(w6) -> (w5:tag[])
  n58 = Unbundle By Name("Test Section Physical Channels") -> ("Evaporator Bottom Temperature"=w4:tag, "Test Section Window 3-4 Pressure"=w2:tag)
  n59 = for {
    tunnel: w101 -> [w540]
    tunnel: w100 -> [w541] mode=indexing
    tunnel: w99 -> [w542] mode=indexing
    tunnel: w98 -> [w530] mode=indexing
    tunnel: w97 -> [w534] mode=indexing
    tunnel: w96 -> [w536] mode=indexing
    tunnel: w5 -> [w535] mode=indexing
    tunnel: [w538] -> w90
    tunnel: w94 -> [w533] mode=indexing
    tunnel: w93 -> [w532] mode=indexing
    tunnel: w92 -> [w531] mode=indexing
    shift-right: [w537] -> w95
    shift-left: w103 -> [w539]
    tunnel: w91 -> [w529] mode=indexing
    n60 = case shown="False" w529 {
      tunnel: w542 -> [w554 w567]
      tunnel: w541 -> [w553 w566]
      tunnel: w540 -> [w552 w565]
      tunnel: w539 -> [w551 w564]
      tunnel: [w550 w563] -> w538
      tunnel: [w549 w562] -> w537
      tunnel: w536 -> [w548 w561]
      tunnel: w535 -> [w547 w560]
      tunnel: w534 -> [w546 w559]
      tunnel: w533 -> [w545 w558]
      tunnel: w532 -> [w544 w557]
      tunnel: w531 -> [w543 w556]
      tunnel: w530 -> [_ w555]
      frame True {
        n61 = call-poly <vilib>:"DAQmx Create Virtual Channel.vi"("task in"=w552, "maximum value"=w554, "minimum value"=w553, "physical channels"=w547, "cjc source"=w545, "name to assign"=w548, "units"=w546, "cjc channel"=w543, "error in"=w551, "cjc value"=w544) -> ("task out"=w550:refnum<k21>, "error out"=w549:errorcluster)  [unwired: 4 in]
      }
      frame False {
        n62 = call-poly <vilib>:"DAQmx Create Virtual Channel.vi"("task in"=w565, "maximum value"=w567, "minimum value"=w566, "physical channels"=w560, "cjc source"=w558, "name to assign"=w561, "units"=w559, "cjc channel"=w556, "error in"=w564, "thermocouple type"=w555, "cjc value"=w557) -> ("task out"=w563:refnum<k21>, "error out"=w562:errorcluster)  [unwired: 3 in]
      }
    }
  }
  n63 = Build Array(w4, w2) -> (w3:tag[])
  n64 = for {
    tunnel: w90 -> [w576]
    tunnel: w89 -> [w577] mode=indexing
    tunnel: w88 -> [w578] mode=indexing
    tunnel: w87 -> [w579] mode=indexing
    tunnel: w86 -> [w569] mode=indexing
    tunnel: w85 -> [w570] mode=indexing
    tunnel: w84 -> [w572] mode=indexing
    tunnel: w3 -> [w571] mode=indexing
    tunnel: [w574] -> w78
    shift-right: [w573] -> w83
    shift-left: w95 -> [w575]
    tunnel: w82 -> [w568] mode=indexing
    n65 = case shown="False" w568 {
      tunnel: w579 -> [w590 w595]
      tunnel: w578 -> [w589 w596]
      tunnel: w577 -> [w588 w597]
      tunnel: w576 -> [w587 w601]
      tunnel: w575 -> [w586 w600]
      tunnel: [w585 w598] -> w574
      tunnel: [w584 w599] -> w573
      tunnel: w572 -> [w583 w593]
      tunnel: w571 -> [w582 w594]
      tunnel: w570 -> [w581 w592]
      tunnel: w569 -> [w580 w591]
      frame False {
        n66 = call-poly <vilib>:"DAQmx Create Virtual Channel.vi"("task in"=w587, "maximum value"=w590, "minimum value"=w589, "input terminal configuration"=w588, "physical channels"=w582, "name to assign"=w583, "units"=w581, "error in"=w586, "custom scale name"=w580) -> ("task out"=w585:refnum<k21>, "error out"=w584:errorcluster)  [unwired: 5 in]
      }
      frame True {
        n67 = call-poly <vilib>:"DAQmx Create Virtual Channel.vi"("task in"=w601, "maximum value"=w595, "minimum value"=w596, "input terminal configuration"=w597, "physical channels"=w594, "name to assign"=w593, "units"=w592, "error in"=w600, "custom scale name"=w591) -> ("task out"=w598:refnum<k21>, "error out"=w599:errorcluster)  [unwired: 5 in]
      }
    }
  }
  n68 = for {
    tunnel: w78 -> [w605]
    tunnel: w81 -> [w606] mode=indexing
    shift-right: [w607] -> w80
    shift-left: w83 -> [w603]
    tunnel: [w604] -> w74
    tunnel: w79 -> [w602] mode=indexing
    tunnel: [w603] -> _ mode=indexing
    n69 = property class="DAQmx Channel"(reference=w605, error in=w603, "Active Channels (if subset)"=w606, "Analog Input:General Properties:Digitizer/ADC:Timing Mode"=w602) -> (reference out=w604:refnum<k21>, error out=w607:errorcluster)
  }
  n70 = for {
    tunnel: w74 -> [w611]
    tunnel: w77 -> [w612] mode=indexing
    shift-right: [w613] -> w76
    shift-left: w80 -> [w609]
    tunnel: [w610] -> w70
    tunnel: w75 -> [w608] mode=indexing
    tunnel: [w609] -> _ mode=indexing
    n71 = property class="DAQmx Channel"(reference=w611, error in=w609, "Active Channels (if subset)"=w612, "AI.AutoZeroMode"=w608) -> (reference out=w610:refnum<k21>, error out=w613:errorcluster)
  }
  n72 = for {
    tunnel: w70 -> [w617]
    tunnel: w73 -> [w618] mode=indexing
    shift-right: [w619] -> w72
    shift-left: w76 -> [w615]
    tunnel: [w616] -> w66
    tunnel: w71 -> [w614] mode=indexing
    tunnel: [w615] -> _ mode=indexing
    n73 = property class="DAQmx Channel"(reference=w617, error in=w615, "Active Channels (if subset)"=w618, "Analog Input:General Properties:Digitizer/ADC:Timing Mode"=w614) -> (reference out=w616:refnum<k21>, error out=w619:errorcluster)
  }
  n74 = for {
    tunnel: w66 -> [w623]
    tunnel: w69 -> [w624] mode=indexing
    shift-right: [w625] -> w68
    shift-left: w72 -> [w621]
    tunnel: [w622] -> w62
    tunnel: w67 -> [w620] mode=indexing
    tunnel: [w621] -> _ mode=indexing
    n75 = property class="DAQmx Channel"(reference=w623, error in=w621, "Active Channels (if subset)"=w624, "AI.AutoZeroMode"=w620) -> (reference out=w622:refnum<k21>, error out=w625:errorcluster)
  }
  n76 = for {
    tunnel: w62 -> [w629]
    tunnel: w65 -> [w630] mode=indexing
    shift-right: [w631] -> w64
    shift-left: w68 -> [w627]
    tunnel: [w628] -> w58
    tunnel: w63 -> [w626] mode=indexing
    tunnel: [w627] -> _ mode=indexing
    n77 = property class="DAQmx Channel"(reference=w629, error in=w627, "Active Channels (if subset)"=w630, "Analog Input:General Properties:Digitizer/ADC:Timing Mode"=w626) -> (reference out=w628:refnum<k21>, error out=w631:errorcluster)
  }
  n78 = for {
    tunnel: w58 -> [w635]
    tunnel: w61 -> [w636] mode=indexing
    shift-right: [w637] -> w60
    shift-left: w64 -> [w633]
    tunnel: [w634] -> w54
    tunnel: w59 -> [w632] mode=indexing
    tunnel: [w633] -> _ mode=indexing
    n79 = property class="DAQmx Channel"(reference=w635, error in=w633, "Active Channels (if subset)"=w636, "AI.AutoZeroMode"=w632) -> (reference out=w634:refnum<k21>, error out=w637:errorcluster)
  }
  n80 = for {
    tunnel: w54 -> [w641]
    tunnel: w57 -> [w642] mode=indexing
    shift-right: [w643] -> w56
    shift-left: w60 -> [w639]
    tunnel: [w640] -> w50
    tunnel: w55 -> [w638] mode=indexing
    tunnel: [w639] -> _ mode=indexing
    n81 = property class="DAQmx Channel"(reference=w641, error in=w639, "Active Channels (if subset)"=w642, "Analog Input:General Properties:Digitizer/ADC:Timing Mode"=w638) -> (reference out=w640:refnum<k21>, error out=w643:errorcluster)
  }
  n82 = for {
    tunnel: w50 -> [w647]
    tunnel: w53 -> [w648] mode=indexing
    shift-right: [w649] -> w52
    shift-left: w56 -> [w645]
    tunnel: [w646] -> w46
    tunnel: w51 -> [w644] mode=indexing
    tunnel: [w645] -> _ mode=indexing
    n83 = property class="DAQmx Channel"(reference=w647, error in=w645, "Active Channels (if subset)"=w648, "AI.AutoZeroMode"=w644) -> (reference out=w646:refnum<k21>, error out=w649:errorcluster)
  }
  n84 = for {
    tunnel: w46 -> [w653]
    tunnel: w49 -> [w654] mode=indexing
    shift-right: [w655] -> w48
    shift-left: w52 -> [w651]
    tunnel: [w652] -> w43
    tunnel: w47 -> [w650] mode=indexing
    tunnel: [w651] -> _ mode=indexing
    n85 = property class="DAQmx Channel"(reference=w653, error in=w651, "Active Channels (if subset)"=w654, "Analog Input:General Properties:Digitizer/ADC:Timing Mode"=w650) -> (reference out=w652:refnum<k21>, error out=w655:errorcluster)
  }
  n86 = call-poly <vilib>:"DAQmx Timing.vi"("task/channels in"=w43, "sample mode"=w42, "samples per channel"="number of samples", "rate"="sampling rate", "error in"=w48) -> ("task out"=→"task out":refnum<k21>, "error out"=→"error out":errorcluster)  [unwired: 9 in]
